vi "State Machine.vi"() -> ()   [LabVIEW 2018]
uses:
  Desktop/Core 1 Exercises_2014/Exercises/Weather Warnings/Weather Data.ctl
panel:
  out "Current Temperature":dbl
  out "Temperature History":dbl[](graph)
  out "Warning":string
  in  "Stop Button":bool
  in  "Lower Limit":dbl
  in  "Upper Limit":dbl=30.0
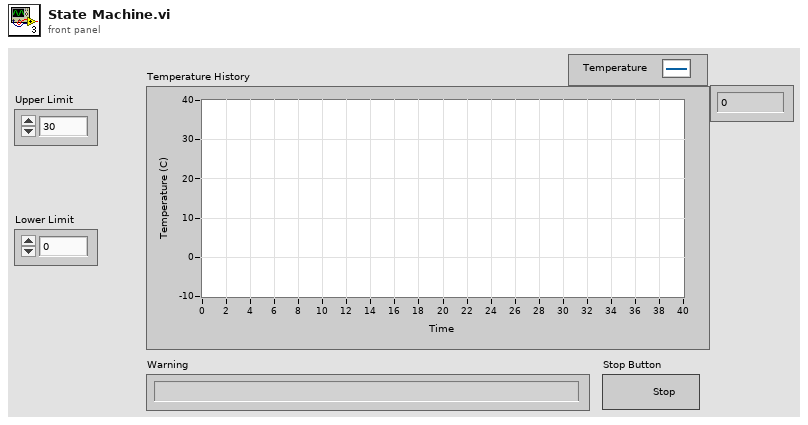
[diagram p1: front panel]
types:
  T1 = enum16{"open", "replace", "create", "open or create", "replace or create", "replace or create with confirmation"}
  T2 = typedef "Weather Data.ctl" = cluster{"Current Temperature":dbl, "Max Temperature":dbl, "Min Temperature":dbl, "Warning?":bool, "Warning Text":string, "Unit":enum16{"Fahrenheit", "Celsius"}}
  T3 = enum16{"Initialize", "Acquisition", "Analysis", "Data Log", "Time check"}
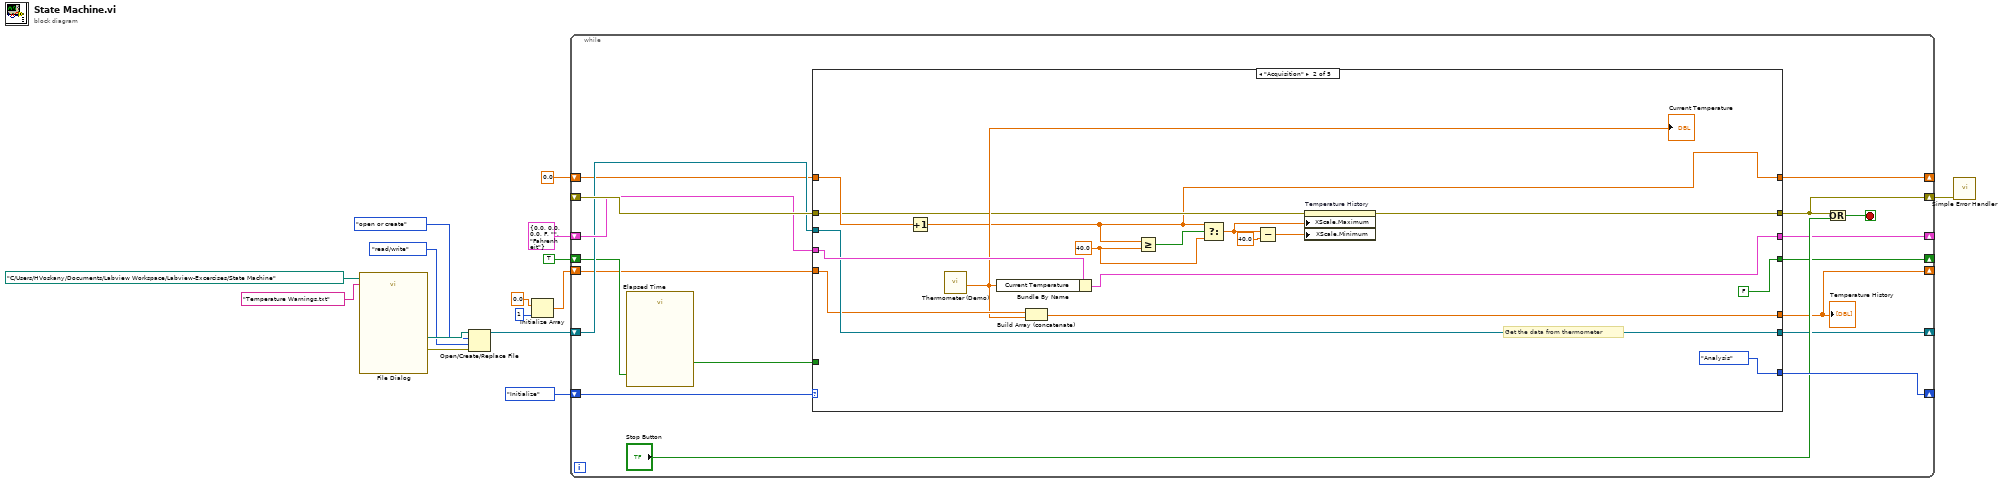
[diagram p0: block diagram]
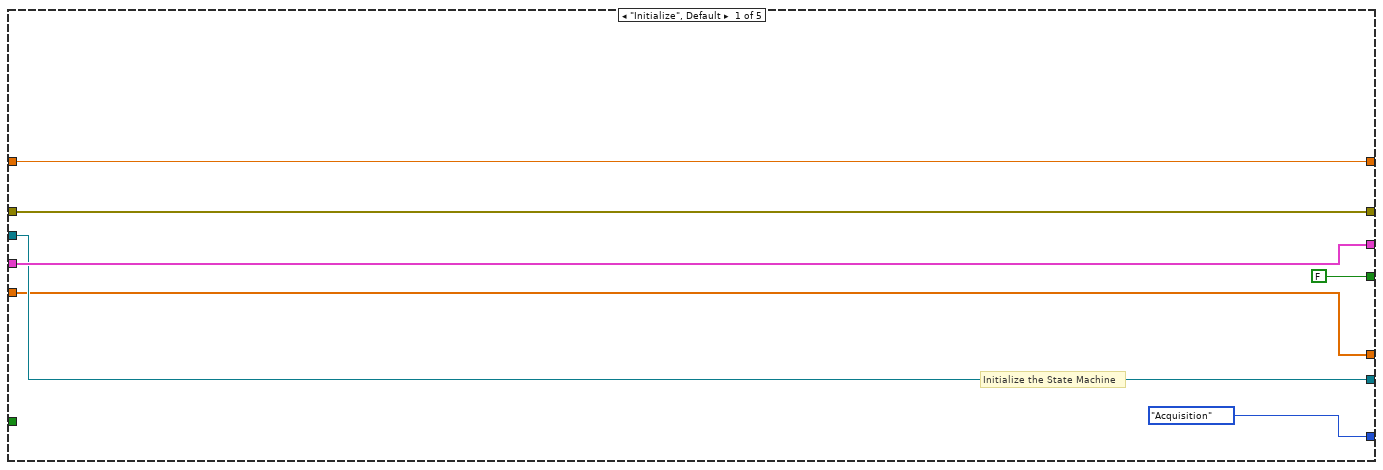
[diagram p2: hidden frame]
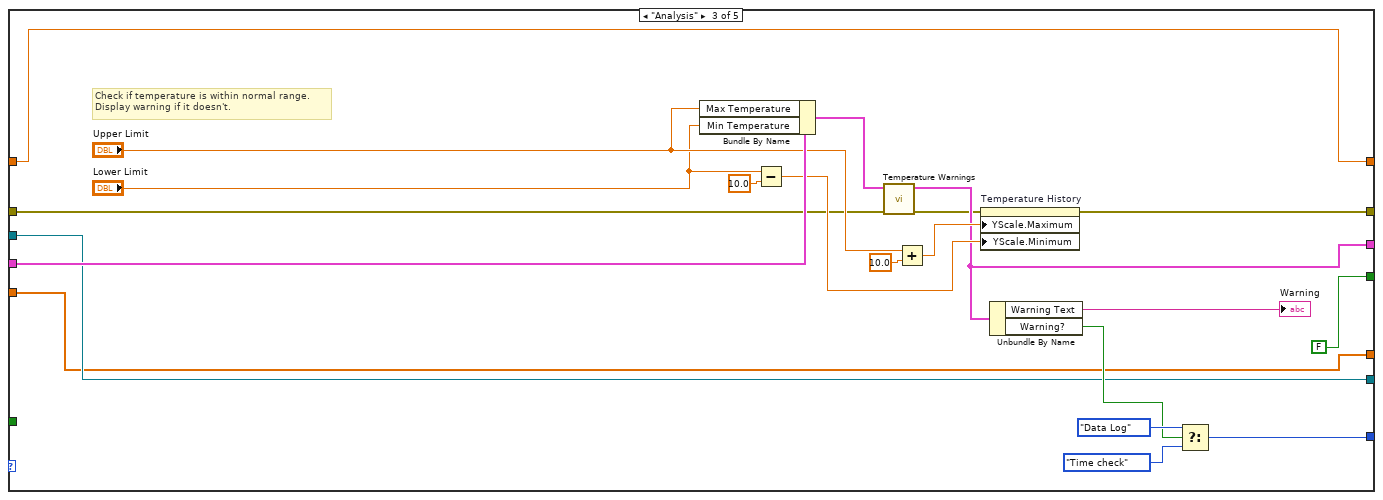
[diagram p3: hidden frame]
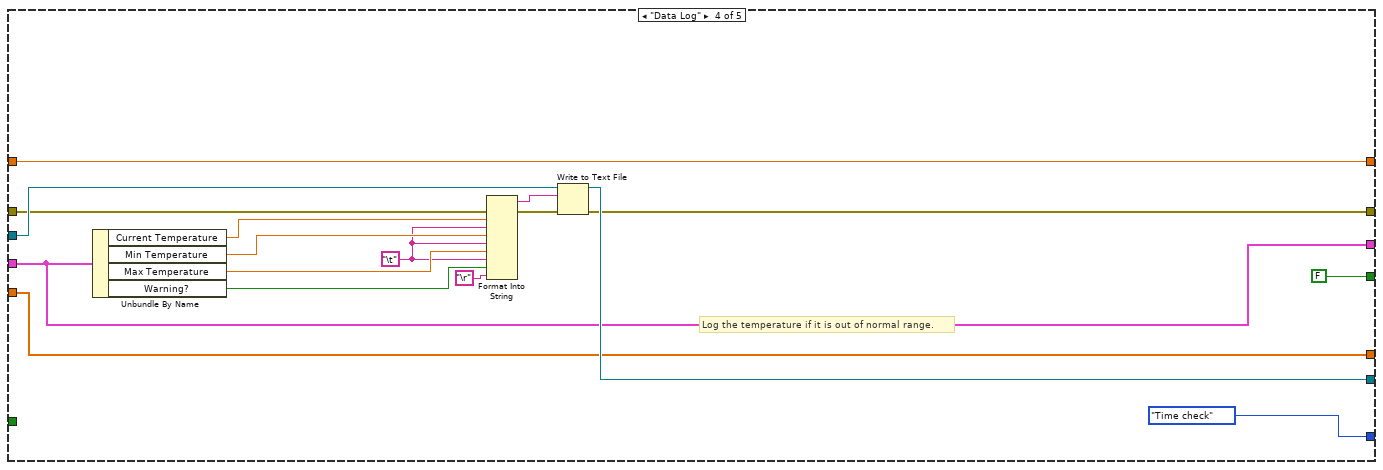
[diagram p4: hidden frame]
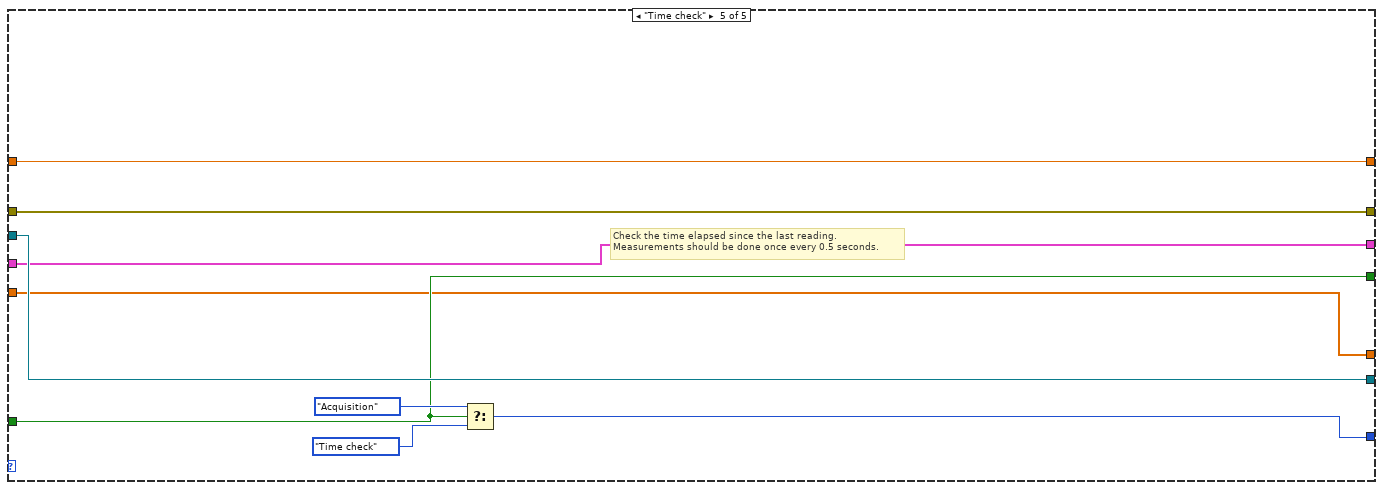
[diagram p5: hidden frame]
diagram:
  n1 = call "File Dialog"("start path"=path "C:/Users/HVoskany/Documents/Labview Workspace/Labview-Excercises/State Machine", "default name"="Temperature Warnings.txt") -> ("selected path"=w9:path, "error out"=w10:errorcluster)  [unwired: 10 in, 2 out]
  n2 = Open/Create/Replace File(file path (use dialog)=w9, error in=w10, operation (0:open)=T1."open or create", access (0:read/write)=enum16{"read/write", "read-only", "write-only"}."read/write") -> (refnum out=w8:refnum<file>)  [unwired: 2 in, 2 out]
  n3 = Initialize Array(0.0 ("element"), 1 ("dimension size")) -> (w2:dbl[])
  n4 = while {
    shift-right: [w30] -> w12
    shift-left: _ -> [w31]
    shift-right: [w27] -> _
    shift-left: T3."Initialize" -> [w29]
    shift-right: [w20] -> _
    shift-left: T2 {"Current Temperature"=0.0, "Max Temperature"=0.0, "Min Temperature"=0.0, "Warning?"=FALSE, "Warning Text"="", "Unit"=enum."Fahrenheit"} ("Weather Data In") -> [w28]
    shift-right: [w24] -> _
    shift-left: w8 -> [w25]
    shift-right: [w21] -> _
    shift-left: TRUE -> [w23]
    shift-right: [w18] -> _
    shift-left: w2 -> [w19]
    shift-right: [w16] -> _
    shift-left: 0.0 -> [w17]
    stop <- w32 stop-if-true
    n5 = call "Elapsed Time"("Reset"=w23) -> ("Time has Elapsed"=w22:bool)  [unwired: 11 in, 7 out]
    n6 = case shown="\"Acquisition\"" w29 {
      tunnel: w28 -> [w38 w55 w77 w91 w101]
      tunnel: w31 -> [w39 w45 w57 w82 w103]
      tunnel: [w39 w44 w67 w92 w103] -> w30
      tunnel: [w38 w54 w59 w91 w101] -> w20
      tunnel: [T3."Acquisition" T3."Analysis" w72 T3."Time check" ("f") w98] -> w27
      tunnel: w25 -> [w36 w53 w71 w94 w102]
      tunnel: [w36 w53 w71 w93 w102] -> w24
      tunnel: w22 -> [_ _ _ _ w97]
      tunnel: [FALSE ("Time has Elapsed") FALSE ("Time has Elapsed") FALSE ("Time has Elapsed") FALSE ("Time has Elapsed") w97] -> w21
      tunnel: w19 -> [w34 w51 w69 w79 w96]
      tunnel: [w34 w49 w69 w79 w96] -> w18
      tunnel: w17 -> [w33 w46 w68 w78 w95]
      tunnel: [w33 w43 w68 w78 w95] -> w16
      frame "Initialize", Default {
        # "Initialize the State Machine"
      }
      frame "Acquisition" {
        w47 = 40.0 ("y")
        # "Get the data from thermometer"
        n7 = Increment(x=w46) -> (x+1=w43:dbl)
        n8 = call "Thermometer (Demo).vi"() -> ("Temperature Value"=w50:dbl)  [unwired: 11 in]
        "Current Temperature" <- w50
        n9 = Bundle By Name(cluster=w55, "Current Temperature"=w50) -> (w54:T2)
        n10 = Build Array (concatenate)(w51, w50) -> (w49:dbl[])
        n11 = Greater Or Equal?(x=w43, y=w47) -> (x >= y?=w48:bool)
        n12 = Select(t=w43, s=w48, f=w47) -> (s? t:f=w42:dbl)
        n13 = Subtract(x=w42, y=40.0) -> (x-y=w40:dbl)
        n14 = property on="Temperature History" class="WFGraph (strict)"(error in=w45, "XScale.Maximum"=w42, "XScale.Minimum"=w40) -> (error out=w44:errorcluster)  [unwired: 1 in, 1 out]
      }
      frame "Analysis" {
        # "Check if temperature is within normal range.\nDisplay warning if it doesn't."
        n15 = Bundle By Name(cluster=w77, "Max Temperature"="Upper Limit", "Min Temperature"="Lower Limit") -> (w60:T2)
        n16 = Subtract(x="Lower Limit", y=10.0) -> (x-y=w61:dbl)
        n17 = call "Temperature Warnings.vi"("Error In"=w57, "Weather Data In"=w60) -> ("Error Out"=w58:errorcluster, "Weather Data Out"=w59:T2)  [unwired: 8 in]
        n18 = Add(x="Upper Limit", y=10.0) -> (x+y=w62:dbl)
        n19 = property on="Temperature History" class="WFGraph (strict)"(error in=w58, "YScale.Maximum"=w62, "YScale.Minimum"=w61) -> (error out=w67:errorcluster)  [unwired: 1 in, 1 out]
        n20 = Unbundle By Name(w59) -> ("Warning Text"=→"Warning":string, "Warning?"=w74:bool)
        n21 = Select(t=T3."Data Log", s=w74, f=T3."Time check") -> (s? t:f=w72:T3)
      }
      frame "Data Log" {
        w85 = "\t"
        # "Log the temperature if it is out of normal range."
        n22 = Unbundle By Name(w91) -> ("Current Temperature"=w88:dbl, "Min Temperature"=w87:dbl, "Max Temperature"=w86:dbl, "Warning?"=w84:bool)
        n23 = Format Into String(error in=w82, w88, w85, w87, w85, w86, w85, w84, "\r") -> (resulting string=w80:string, error out=w81:errorcluster)  [unwired: 2 in]
        n24 = Write to Text File(file (use dialog)=w94, text=w80, error in=w81) -> (refnum out=w93:refnum<file>, error out=w92:errorcluster)  [unwired: 1 in, 1 out]
      }
      frame "Time check" {
        # "Check the time elapsed since the last reading.\nMeasurements should be done once every 0.5 seconds."
        n25 = Select(t=T3."Acquisition", s=w97, f=T3."Time check") -> (s? t:f=w98:T3)
      }
    }
    "Temperature History" <- w18
    n26 = Or(x=w30, y="Stop Button") -> (x .or. y?=w32:bool)
  }
  n27 = call <vilib>:"Simple Error Handler.vi"("error in (no error)"=w12) -> ()  [unwired: 4 in, 5 out]
